vi "Complex LU Linear Equations.vi"(2 "Known Vector":cdb[](array[numeric]) format="%.2f", 3 "LU Info":cluster{"LU":cdb[][], "Pivot":i32[]} {"LU" format="%.3f"}) -> (0 "error":i32, 1 "Solution Vector":cdb[](array[numeric]) format="%.2f")   [LabVIEW 2014, in "NI_AALBase.lvlib"]
doc: "Solves a linear system of simultaneous equations, if possible. The system is solved using the method known as L-U decomposition."
uses:
  NI_AALBase.lvlib
  lvanlys.dll
panel:
  # "Complex LU Linear Equations"
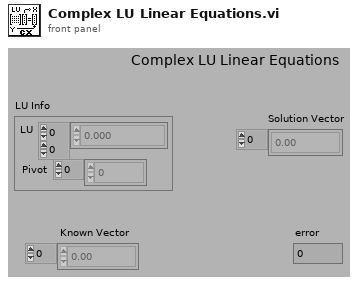
[diagram p1: front panel]
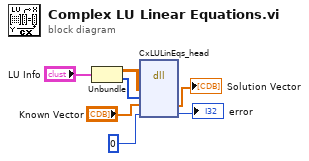
[diagram p0: block diagram]
diagram:
  n1 = Unbundle("LU Info") -> ("LU"=w6:cdb[][], "Pivot"=w5:i32[])
  n2 = dll-call lib="C:/Program Files (x86)/National Instruments/LabVIEW 2014/resource/lvanlys.*" fn="CxLULinEqs_head"("LU"=w6, "Pivot"=w5, "Known Vector"="Known Vector", 0) -> ("Known Vector"=→"Solution Vector":cdb[], →"error":i32)  [unwired: 6 in, 2 out]
